vi "Execute.vi"(8 "error in (no error)":errorcluster, 10 "Abstract Consumer in":refnum<class "Abstract Consumer.lvclass">, 11 "Shutdown Message in":refnum<class "Shutdown Message.lvclass">) -> (0 "error out":errorcluster, 1 "Abstract Response out":refnum<class "Abstract Response Message.lvclass">, 2 "Abstract Consumer out":refnum<class "Abstract Consumer.lvclass">, 3 "Shutdown Message out":refnum<class "Shutdown Message.lvclass">, 4 "Stop?":bool)   [LabVIEW 2017, in "Messaging.lvlib" / "Shutdown Message.lvclass"]
uses:
  Shutdown Message.lvclass
  Consumer/Abstract Consumer/Abstract Consumer.lvclass
  Abstract Response Message/Abstract Response Message.lvclass
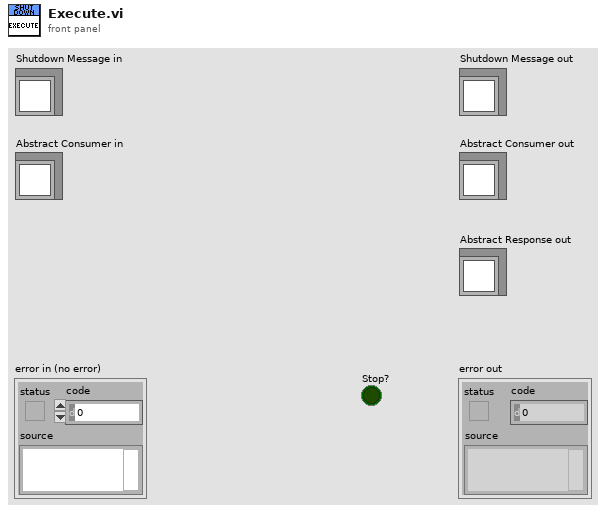
[diagram p1: front panel]
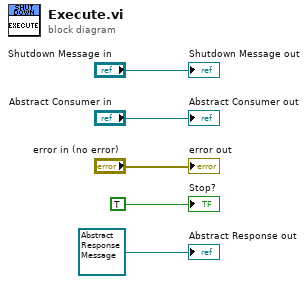
[diagram p0: block diagram]
diagram:
  "error out" <- "error in (no error)"
  "Shutdown Message out" <- "Shutdown Message in"
  "Abstract Consumer out" <- "Abstract Consumer in"
  "Stop?" <- TRUE ("Stop?")
  "Abstract Response out" <- refnum<class "Abstract Response Message.lvclass"> refnum ("Abstract Response out")
